vi "Main.InitializeXNET.vi"(7 "Name":string, 8 "error in (no error)":errorcluster, 9 "PCL":u32, 10 "Data Settings":T19 {"Monitor"."Data"."Outgoing"."Trigger.Refs"."Data Reference" format="%.0x"; "Monitor"."Data"."Outgoing"."Disable.Refs"."Data Reference" format="%.0x"; "Monitor"."Data"."Outgoing"."Data.Refs"."Data Reference" format="%.0x"; "Monitor"."Data"."Incoming"."Timing.Refs"."Data Reference" format="%.0x"; "Monitor"."Data"."Incoming"."Data.Refs"."Data Reference" format="%.0x"; "Monitor"."Network"."Name" format="%.0x"; "Sim"."DTCs"."DM1.Ref"."Data Reference" format="%.0x"; "Sim"."DTCs"."DM1.Enable.Ref"."Data Reference" format="%.0x"; "Sim"."DTCs"."DM2.Ref"."Data Reference" format="%.0x"; "Sim"."DTCs"."DM2.Enable.Ref"."Data Reference" format="%.0x"; "Sim"."Network"."Name" format="%.0x"}, 11 "XNET Settings":T2 {"Termination" items=["Off", "On"]}) -> (0 "error out":errorcluster, 3 "Protocol App":T1={"Name"="", "XNET.Settings"={"Database"="", "Cluster"="", "Port"="", "Baud rate [Bd]"=0, "Termination"=0, "Incoming Decimation"=0, "Outgoing Decimation"=1}, "Monitor.Network"={"Address"=0, "Name"=0, "Include DA"=FALSE, "Force SA"=FALSE}, "Data"=[], "DTCs"=[], "Sim.Nodes.LUT"=variant, "Data.LUT"=variant, "PCL"=0} {"Monitor.Network"."Name" format="%.0x"; "DTCs"."Data"."DM1.Ref"."Data Reference" format="%.0x"; "DTCs"."Data"."DM1.Enable.Ref"."Data Reference" format="%.0x"; "DTCs"."Data"."DM2.Ref"."Data Reference" format="%.0x"; "DTCs"."Data"."DM2.Enable.Ref"."Data Reference" format="%.0x"; "Data"."Trigger.Refs"."Data Reference" format="%.0x"; "Data"."Disable.Refs"."Data Reference" format="%.0x"; "Data"."Timing.Refs"."Data Reference" format="%.0x"; "Data"."Network"."Name" format="%.0x"; "Data"."Incoming.Refs"."Data Reference" format="%.0x"; "Data"."Outgoing.Refs"."Data Reference" format="%.0x"; "XNET.Settings"."Termination" items=["Off", "On"]})   [LabVIEW 2023, in "J1939 Addon Engine.lvlib"]
uses:
  J1939 Addon Engine.lvlib
  Addon Shared/Types/XNET Settings.ctl
  Addon Shared/Types/Compiled.Node Settings.ctl
  Addon Shared/Types/Compiled Monitor Tool Settings.ctl
  Addon Shared/Types/Monitor Settings.ctl
  Addon Shared/Types/Device Settings.ctl
  Addon Shared/Types/Incoming Settings.ctl
  Addon Shared/Types/Incoming Frame Settings.ctl
  <vilib>/NI VeriStand/Custom Device API/Block Data Reference.ctl
  <vilib>/NI VeriStand/Custom Device API/Data Reference.ctl
  Addon Shared/Types/Outgoing Settings.ctl
  Addon Shared/Types/Outgoing Frame Settings.ctl
  Addon Shared/Types/Outgoing Event Trigger Types.ctl
  SubModules/Frame-Protection-Support/Source/Shared/Types/Exported Frame Settings.ctl
  SubModules/Frame-Protection-Support/Source/Shared/Types/Exported Frame Type.ctl
  SubModules/Frame-Protection-Support/Source/Shared/Types/Exported Protection Settings.ctl
  SubModules/Frame-Protection-Support/Source/Shared/Types/Protection Type.ctl
  SubModules/Frame-Protection-Support/Source/Shared/Types/XNET Signal Configuration.ctl
  SubModules/Frame-Protection-Support/Source/Shared/Types/Exported Counter Settings.ctl
  SubModules/Frame-Protection-Support/Source/Shared/Types/Exported Event Trigger Type.ctl
  Addon Shared/Types/Complied Simulated Device Settings.ctl
  Addon Shared/Types/Compiled Simulated Settings.ctl
  Types/Protocol.App Settings.ctl
  Types/Protocol.XNET Refs.ctl
  Types/Main.Outgoing.Frame.Settings.ctl
  Types/Engine.DTC Settings.ctl
  Types/Engine.DTC FIFOs.ctl
  Types/Engine.Node DTC Settings.ctl
  Addon Shared/J1939 Addon Shared.lvlib
  <vilib>/NI VeriStand/Custom Device API/Custom Device API.lvlib
  SubModules/Frame-Protection-Support/Source/Shared/Protection and Counter Support Shared.lvlib
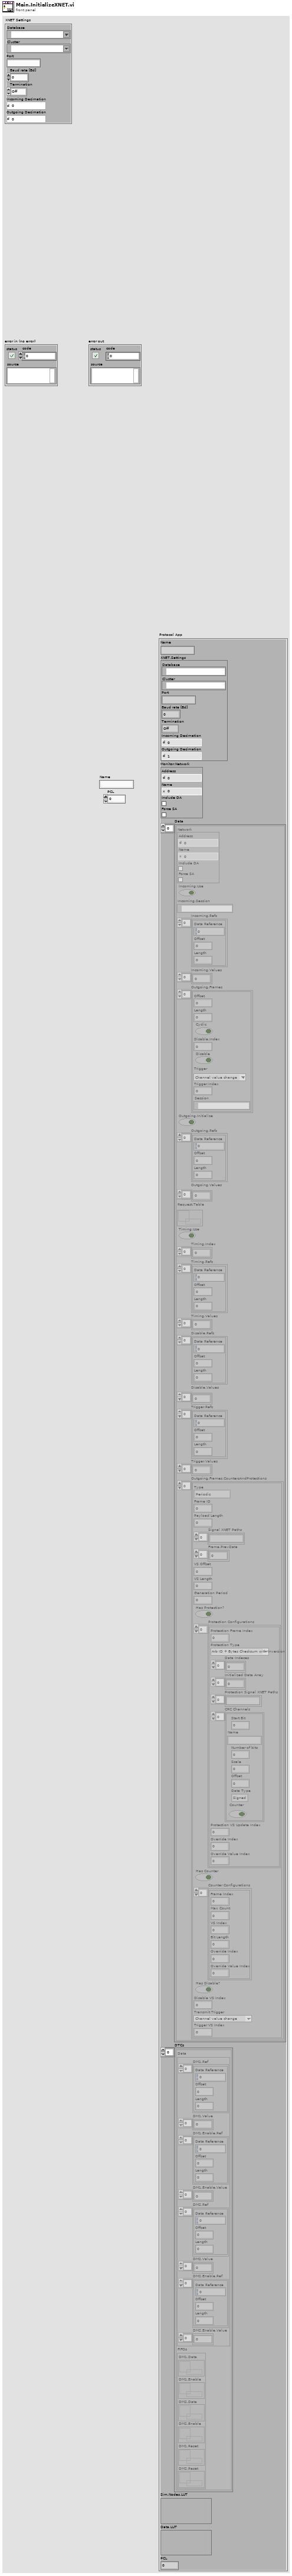
[diagram p1: front panel]
types:
  T1 = typedef "J1939 Addon Engine.lvlib/Protocol.App Settings.ctl" = cluster{"Name":string, "XNET.Settings":T2, "Monitor.Network":T3, "Data":T4[], "DTCs":T16[], "Sim.Nodes.LUT":variant, "Data.LUT":variant, "PCL":u32}
  T2 = typedef "J1939 Addon Shared.lvlib/XNET Settings.ctl" = cluster{"Database":refnum<k21>, "Cluster":refnum<k21>, "Port":string, "Baud rate [Bd]":u32, "Termination":u32, "Incoming Decimation":u32, "Outgoing Decimation":u32}
  T3 = typedef "J1939 Addon Shared.lvlib/Monitor Settings.ctl" = cluster{"Address":u8, "Name":u64, "Include DA":bool, "Force SA":bool}
  T4 = typedef "J1939 Addon Engine.lvlib/Protocol.XNET Refs.ctl" = cluster{"Network":T3, "Incoming.Use":bool, "Incoming.Session":refnum<k21>, "Incoming.Refs":T5[], "Incoming.Values":dbl[], "Outgoing.Frames":T7[], "Outgoing.Initialize":bool, "Outgoing.Refs":T5[], "Outgoing.Values":dbl[], "Request.Table":refnum<k33>, "Timing.Use":bool, "Timing.Index":i32[], "Timing.Refs":T5[], "Timing.Values":dbl[], "Disable.Refs":T5[], "Disable.Values":dbl[], "Trigger.Refs":T5[], "Trigger.Values":dbl[], "Outgoing.Frames.CountersAndProtections":T9[]}
  T5 = typedef "Custom Device API.lvlib/Block Data Reference.ctl" = cluster{"Data Reference":T6, "Offset":u64, "Length":u64}
  T6 = typedef "Custom Device API.lvlib/Data Reference.ctl" = i32
  T7 = typedef "J1939 Addon Engine.lvlib/Main.Outgoing.Frame.Settings.ctl" = cluster{"Offset":u32, "Length":u32, "Cyclic":bool, "Disable.Index":i32, "Disable":bool, "Trigger":T8, "Trigger.Index":i32, "Session":refnum<k21>}
  T8 = typedef "J1939 Addon Shared.lvlib/Outgoing Event Trigger Types.ctl" = enum16{"Channel value change", "Trigger channel (not zero)", "Channel value change or trigger channel (not zero)", "Trigger channel (any value change)", "Channel value change or trigger channel (any value change)"}
  T9 = typedef "Protection and Counter Support Shared.lvlib/Exported Frame Settings.ctl" = cluster{"Type":T10, "Frame ID":u32, "Payload Length":u32, "Signal XNET Paths":string[], "Frame.PrevData":dbl[], "VS Offset":i32, "VS Length":i32, "Generation Period":u32, "Has Protection?":bool, "Protection Configurations":T11[], "Has Counter":bool, "Counter Configurations":T14[], "Has Disable?":bool, "Disable VS Index":i32, "Transmit Trigger":T15, "Trigger VS Index":i32}
  T10 = typedef "Protection and Counter Support Shared.lvlib/Exported Frame Type.ctl" = enum16{"Periodic", "Event", "Periodic/Event"}
  T11 = typedef "Protection and Counter Support Shared.lvlib/Exported Protection Settings.ctl" = cluster{"Protection Frame Index":i32, "Protection Type":T12, "Data Indeces":i32[], "Initialized Data Array":dbl[], "Protection Signal XNET Paths":string[], "CRC Channels":T13[], "Protection VS Update Index":i32, "Override Index":i32, "Override Value Index":i32}
  T12 = typedef "Protection and Counter Support Shared.lvlib/Protection Type.ctl" = enum16{"Arb ID + Bytes Checksum with Inversion", "Arb ID + Bytes CRC with Inversion", "Reversed Raw Signal Checksum with Inversion", "Concatenated Two's Compliment"}
  T13 = typedef "Protection and Counter Support Shared.lvlib/XNET Signal Configuration.ctl" = cluster{"Start Bit":i32, "Name":string, "Number of bits":i32, "Scale":dbl, "Offset":dbl, "Data Type":u32, "Counter":bool}
  T14 = typedef "Protection and Counter Support Shared.lvlib/Exported Counter Settings.ctl" = cluster{"Frame Index":i32, "Max Count":dbl, "VS Index":i32, "Bit Length":i64, "Override Index":i32, "Override Value Index":i32}
  T15 = typedef "Protection and Counter Support Shared.lvlib/Exported Event Trigger Type.ctl" = enum16{"Channel value change", "Trigger channel (not zero)", "Channel value change or trigger channel (not zero)", "Trigger channel (any value change)", "Channel value change or trigger channel (any value change)"}
  T16 = typedef "J1939 Addon Engine.lvlib/Engine.DTC Settings.ctl" = cluster{"Data":T17, "FIFOs":T18}
  T17 = typedef "J1939 Addon Shared.lvlib/Compiled Simulated Settings.ctl" = cluster{"DM1.Ref":T5[], "DM1.Value":dbl[], "DM1.Enable.Ref":T5[], "DM1.Enable.Value":dbl[], "DM2.Ref":T5[], "DM2.Value":dbl[], "DM2.Enable.Ref":T5[], "DM2.Enable.Value":dbl[]}
  T18 = typedef "J1939 Addon Engine.lvlib/Engine.DTC FIFOs.ctl" = cluster{"DM1.Data":refnum<k33>, "DM1.Enable":refnum<k33>, "DM2.Data":refnum<k33>, "DM2.Enable":refnum<k33>, "DM1.Reset":refnum<k33>, "DM2.Reset":refnum<k33>}
  T19 = typedef "J1939 Addon Shared.lvlib/Compiled.Node Settings.ctl" = cluster{"Monitor":T20, "Sim":T26[]}
  T20 = typedef "J1939 Addon Shared.lvlib/Compiled Monitor Tool Settings.ctl" = cluster{"Network":T3, "Data":T21}
  T21 = typedef "J1939 Addon Shared.lvlib/Device Settings.ctl" = cluster{"Incoming":T22, "Outgoing":T24}
  T22 = typedef "J1939 Addon Shared.lvlib/Incoming Settings.ctl" = cluster{"Signals":string[], "Frames":T23[], "Data.Refs":T5[], "Data.Values":dbl[], "Timing.Use":bool, "Timing.Refs":T5[], "Timing.Values":dbl[], "Timing.Index":i32[]}
  T23 = typedef "J1939 Addon Shared.lvlib/Incoming Frame Settings.ctl" = cluster{"Signals":string[], "PGN":u32}
  T24 = typedef "J1939 Addon Shared.lvlib/Outgoing Settings.ctl" = cluster{"Frames":T25[], "Data.Refs":T5[], "Data.Values":dbl[], "Disable.Refs":T5[], "Disable.Values":dbl[], "Trigger.Refs":T5[], "Trigger.Values":dbl[], "Frames.CountersAndProtections":T9[]}
  T25 = typedef "J1939 Addon Shared.lvlib/Outgoing Frame Settings.ctl" = cluster{"Signals":string[], "Channel Array Position":cluster{"Offset":u32, "Length":u32}, "PGN":u32, "Cyclic?":bool, "Disable?":bool, "Disable.Index":i32, "Trigger":T8, "Trigger.Index":i32}
  T26 = typedef "J1939 Addon Shared.lvlib/Complied Simulated Device Settings.ctl" = cluster{"Network":T3, "Data":T21, "DTCs":T17}
  T27 = typedef "J1939 Addon Engine.lvlib/Engine.Node DTC Settings.ctl" = cluster{"Network":T3, "Sim DTC Refs":T16}
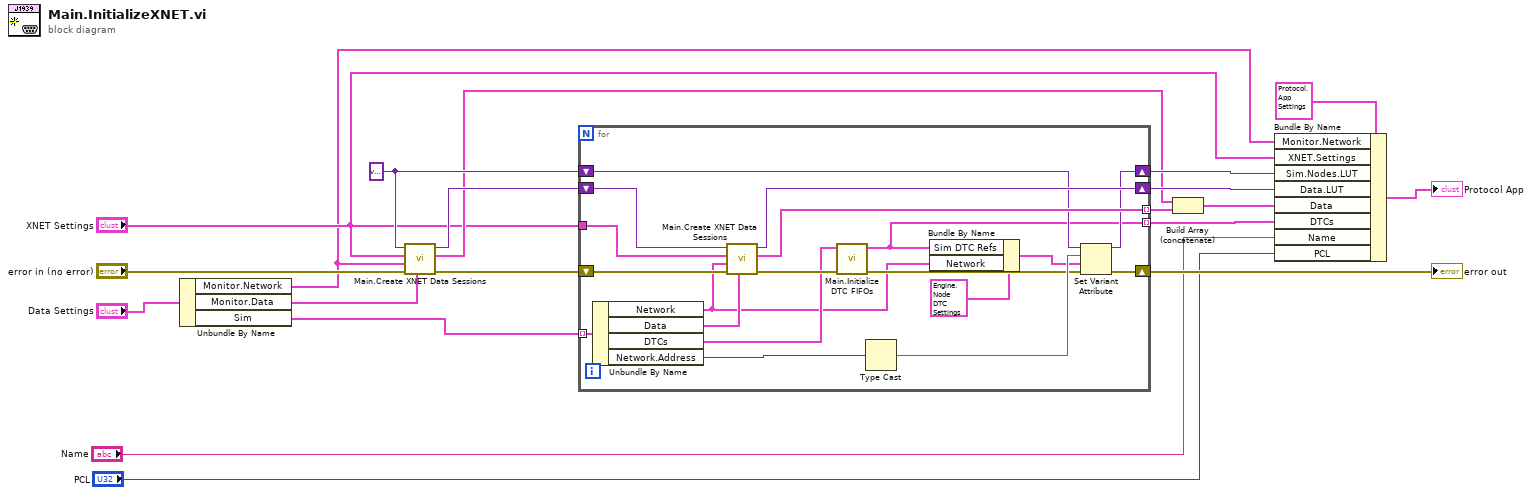
[diagram p0: block diagram]
diagram:
  w15 = variant ("variant")
  n1 = Unbundle By Name("Data Settings") -> ("Monitor.Network"=w2:T3, "Monitor.Data"=w13:T21, "Sim"=w18:T26[])
  n2 = call "Main.Create XNET Data Sessions.vi"("Data"=w13, "error in (no error)"="error in (no error)", "Network"=w2, "J1939 XNET Settings"="XNET Settings", "DataTableLUT"=w15) -> ("error out"=w5:errorcluster, "XNET Sessions"=w6:T4, "DataTableLUT"=w14:variant)  [unwired: 4 in]
  n3 = for {
    tunnel: w18 -> [w35] mode=indexing
    tunnel: "XNET Settings" -> [w36]
    shift-right: [w27] -> w17
    shift-left: w5 -> [w39]
    tunnel: [w38] -> w20 mode=indexing
    shift-right: [w29] -> w9
    shift-left: w14 -> [w33]
    shift-right: [w25] -> w8
    shift-left: w15 -> [w26]
    tunnel: [w24] -> w10 mode=indexing
    n4 = Unbundle By Name(w35) -> ("Network"=w21:T3, "Data"=w34:T21, "DTCs"=w32:T17, "Network.Address"=w30:u8)
    n5 = call "Main.Create XNET Data Sessions.vi"("Data"=w34, "error in (no error)"=w39, "Network"=w21, "J1939 XNET Settings"=w36, "DataTableLUT"=w33) -> ("error out"=w37:errorcluster, "XNET Sessions"=w38:T4, "DataTableLUT"=w29:variant)  [unwired: 4 in]
    n6 = call "Main.Initialize DTC FIFOs.vi"("error in"=w37, "Sim DTCs"=w32) -> ("error out"=w28:errorcluster, "Sim DTC Refs"=w24:T16)  [unwired: 8 in]
    n7 = Type Cast(x=w30) -> (*(type *) &x=w31:string)  [unwired: 1 in]
    n8 = Bundle By Name(cluster=T27 {"Network"={"Address"=0, "Name"=0, "Include DA"=FALSE, "Force SA"=FALSE}, "Sim DTC Refs"={"Data"={"DM1.Ref"=[], "DM1.Value"=[], "DM1.Enable.Ref"=[], "DM1.Enable.Value"=[], "DM2.Ref"=[], "DM2.Value"=[], "DM2.Enable.Ref"=[], "DM2.Enable.Value"=[]}, "FIFOs"={"DM1.Data"=refnum, "DM1.Enable"=refnum, "DM2.Data"=refnum, "DM2.Enable"=refnum, "DM1.Reset"=refnum, "DM2.Reset"=refnum}}}, "Sim DTC Refs"=w24, "Network"=w21) -> (w23:T27)
    n9 = Set Variant Attribute(Variant=w26, name=w31, value=w23, error in=w28) -> (Variant out=w25:variant, error out=w27:errorcluster)  [unwired: 1 out]
  }
  "error out" <- w17
  n10 = Build Array (concatenate)(w6, w20) -> (w11:T4[])
  n11 = Bundle By Name(cluster=T1 {"Name"="", "XNET.Settings"={"Database"="", "Cluster"="", "Port"="", "Baud rate [Bd]"=0, "Termination"=0, "Incoming Decimation"=0, "Outgoing Decimation"=1}, "Monitor.Network"={"Address"=0, "Name"=0, "Include DA"=FALSE, "Force SA"=FALSE}, "Data"=[], "DTCs"=[], "Sim.Nodes.LUT"=variant, "Data.LUT"=variant, "PCL"=0} ("Protocol App"), "Monitor.Network"=w2, "XNET.Settings"="XNET Settings", "Sim.Nodes.LUT"=w8, "Data.LUT"=w9, "Data"=w11, "DTCs"=w10, "Name"="Name", "PCL"="PCL") -> (→"Protocol App":T1)
